vi "Write Count.vi"(8 "error in (no error)":errorcluster, 10 "Count":u32, 11 "Count Response Message in":refnum<class "Count Response Message.lvclass">) -> (0 "error out":errorcluster, 3 "Count Response Message out":refnum<class "Count Response Message.lvclass">)   [LabVIEW 2027, in "Count Response Message.lvclass"]
uses:
  Count Response Message.lvclass
  Count Response Message.lvclass/Count Response Message.ctl
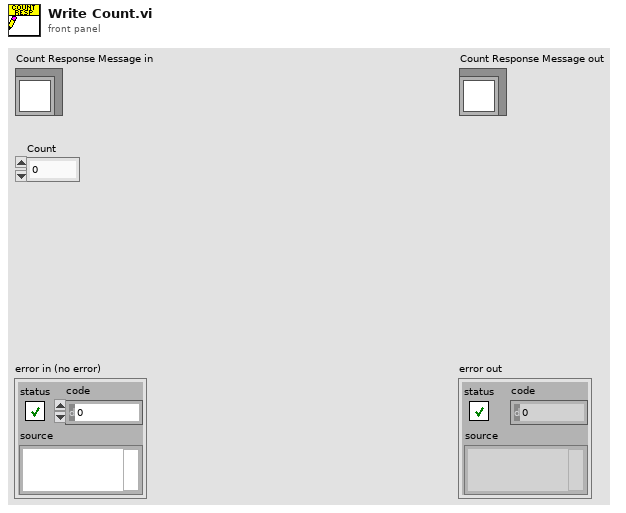
[diagram p1: front panel]
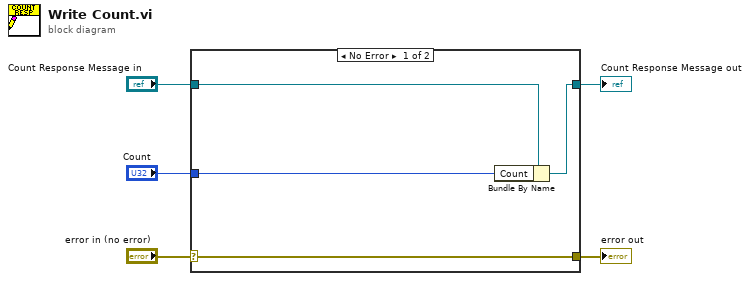
[diagram p0: block diagram]
diagram:
  n1 = case shown="No Error" "error in (no error)" {
    selector: "error in (no error)" -> [w9 w10]
    tunnel: [w9 w10] -> w4
    tunnel: [w7 w11] -> w2
    tunnel: "Count Response Message in" -> [w8 w11]
    tunnel: "Count" -> [w6 _]
    frame No Error {
      n2 = Bundle By Name(cluster=w8, "Count"=w6) -> (w7:refnum<class "Count Response Message.lvclass">)
    }
    frame Error {
    }
  }
  "error out" <- w4
  "Count Response Message out" <- w2
